vi "Array_Subset by indexes.vi"(0 "Array in":dbl[](array[numeric])=[0.0, 1.0, 2.0, 3.0, 4.0], 1 "Start point index":i32, 2 "End point index":i32=3) -> (14 "Array out":dbl[](array[numeric]))   [LabVIEW 2020]
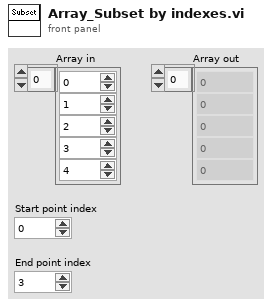
[diagram p1: front panel]
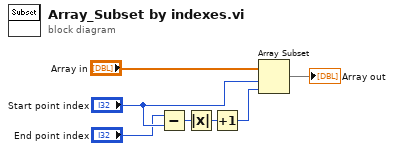
[diagram p0: block diagram]
diagram:
  n1 = Subtract(x="End point index", y="Start point index") -> (x-y=w3:i32)
  n2 = Absolute Value(x=w3) -> (abs(x)=w4:i32)
  n3 = Increment(x=w4) -> (x+1=w5:i32)
  n4 = Array Subset "Array Subset"(array="Array in", index="Start point index", length=w5) -> (→"Array out":dbl[])
